vi "myRIO_BRig_FPGA_stateSelection__v2.vi"(0 "I_selectionState":bool, 2 "I_selectRight":bool, 3 "I_selectWrong":bool, 5 "I_Left(F)_or_Right(T)":bool, 6 "I_ignoreWrong":bool, 8 "I_lickL":bool, 10 "I_lickR":bool) -> (22 "output__I_selectRight":bool, 23 "output__I_selectWrong":bool)   [LabVIEW 2014]
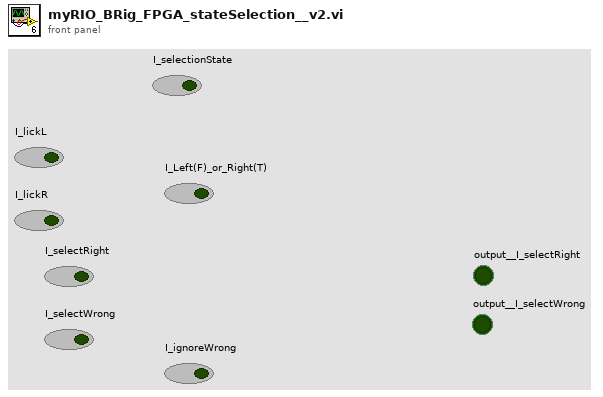
[diagram p1: front panel]
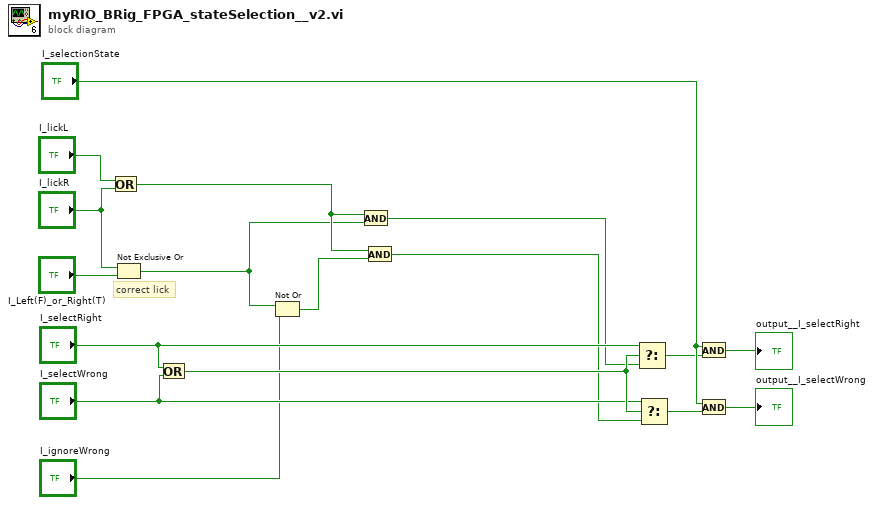
[diagram p0: block diagram]
diagram:
  # "correct lick"
  n1 = Or(x="I_lickL", y="I_lickR") -> (x .or. y?=w3:bool)
  n2 = Not Exclusive Or(1:"I_Left(F)_or_Right(T)", 2:"I_lickR") -> (0:w2:bool)
  n3 = Or(x="I_selectRight", y="I_selectWrong") -> (x .or. y?=w10:bool)
  n4 = Not Or(1:"I_ignoreWrong", 2:w2) -> (0:w5:bool)
  n5 = And(x=w3, y=w2) -> (x .and. y?=w1:bool)
  n6 = And(x=w3, y=w5) -> (x .and. y?=w4:bool)
  n7 = Select(t="I_selectRight", s=w10, f=w1) -> (s? t:f=w7:bool)
  n8 = Select(t="I_selectWrong", s=w10, f=w4) -> (s? t:f=w11:bool)
  n9 = And(x="I_selectionState", y=w7) -> (x .and. y?=→"output__I_selectRight":bool)
  n10 = And(x="I_selectionState", y=w11) -> (x .and. y?=→"output__I_selectWrong":bool)
